vi "Client Vision TS.vi"(10 "Channel Number":i32, 11 "Address":string) -> (0 "error out":errorcluster)   [LabVIEW 2026]
uses:
  labview/auto-vision/Automotive Vision UI/Automotive-Vision-OOBService_client/RPC Messages/hwval_ExportRequest.ctl
  labview/auto-vision/Automotive Vision UI/Automotive-Vision-OOBService_client/Automotive-Vision-OOBService_client.lvlib
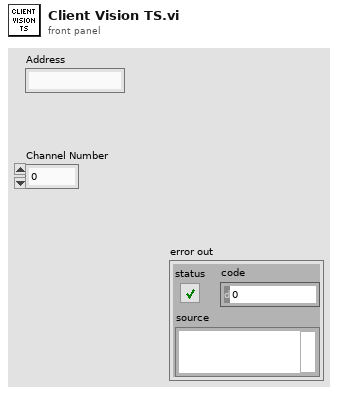
[diagram p1: front panel]
types:
  T1 = typedef "Automotive-Vision-OOBService_client.lvlib/hwval_ExportRequest.ctl" = cluster{"FilePath":string}
  T2 = typedef "grpc-lvsupport-release.lvlib/grpcId.ctl" = u64
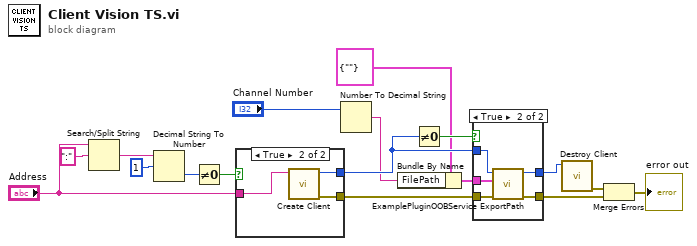
[diagram p0: block diagram]
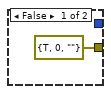
[diagram p3: hidden frame]
diagram:
  n1 = Search/Split String(string="Address", search string/char (-)=":") -> (match + rest of string=w6:string)  [unwired: 1 in, 2 out]
  n2 = Decimal String To Number(string=w6, offset=1) -> (number=w8:i32)  [unwired: 1 in, 1 out]
  n3 = Not Equal To 0?(x=w8) -> (x != 0?=w17:bool)
  n4 = case shown="True" w17 {
    tunnel: [errorcluster {"status"=TRUE, "code"=0, "source"=""} ("error out") w20] -> w16
    tunnel: [_ w21] -> w15
    tunnel: "Address" -> [_ w19]
    frame False {
    }
    frame True {
      n5 = call "Create Client.vi"("address"=w19) -> ("error out"=w20:errorcluster, "gRPC ID Out"=w21:T2)  [unwired: 9 in]
    }
  }
  n6 = Number To Decimal String(number="Channel Number") -> (decimal integer string=w1:string)  [unwired: 1 in]
  n7 = Bundle By Name(cluster=T1 {"FilePath"=""} ("Request Data"), "FilePath"=w1) -> (w5:T1)
  n8 = Not Equal To 0?(x=w15) -> (x != 0?=w4:bool)
  n9 = case shown="True" w4 {
    tunnel: [w23 w25] -> w14
    tunnel: [w22 w27] -> w11
    tunnel: w15 -> [w23 w26]
    tunnel: w16 -> [w22 w28]
    tunnel: w5 -> [_ w24]
    frame False {
    }
    frame True {
      n10 = call "ExamplePluginOOBService ExportPath.vi"("error in"=w28, "Request Data"=w24, "gRPC ID"=w26) -> ("error out"=w27:errorcluster, "gRPC ID out"=w25:T2)  [unwired: 6 in, 1 out]
    }
  }
  n11 = call "Destroy Client.vi"("gRPC ID"=w14) -> ("error out"=w13:errorcluster)  [unwired: 10 in]
  n12 = Merge Errors(w13, w11) -> (→"error out":errorcluster)
